vi "點檢_雷射_命令(切圓)VI.vi"(7 "半徑":dbl min=0.0 max=999.0, 8 "error in (no error)":errorcluster, 9 "雷射圓心座標":cluster{"X":dbl, "Y":dbl} {"X" min=0.0 max=220.0}, 10 "掃描速率(刀速)":u16=220 max=2000 format="%0.0f", 11 "功率":u8=70 max=80) -> (0 "error out":errorcluster, 3 "命令字串":string)   [LabVIEW 2015]
panel:
  out "Y座標":string
  out "x座標":string
  out "命令Array":string[](array[string])
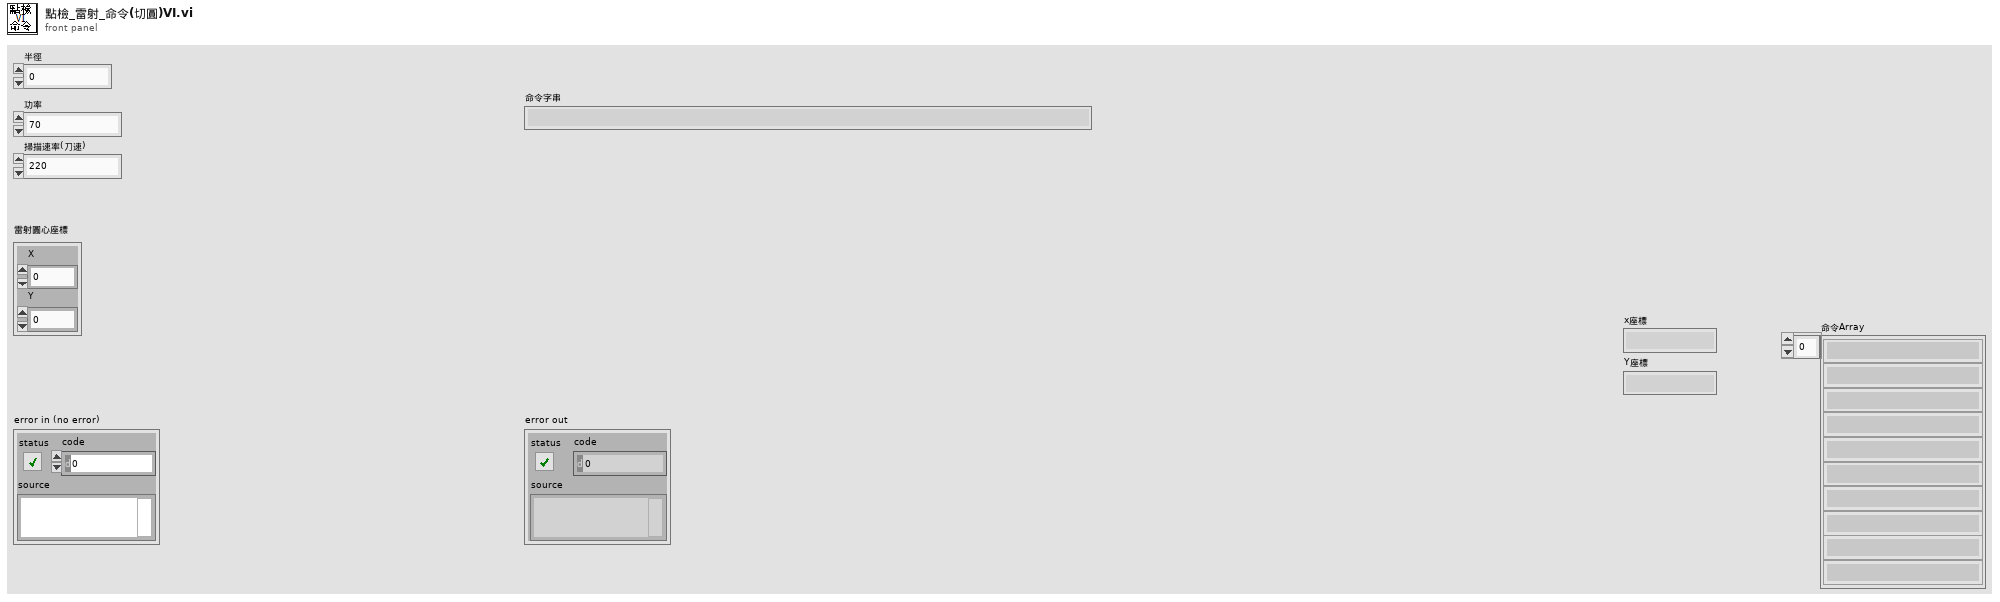
[diagram p1: front panel]
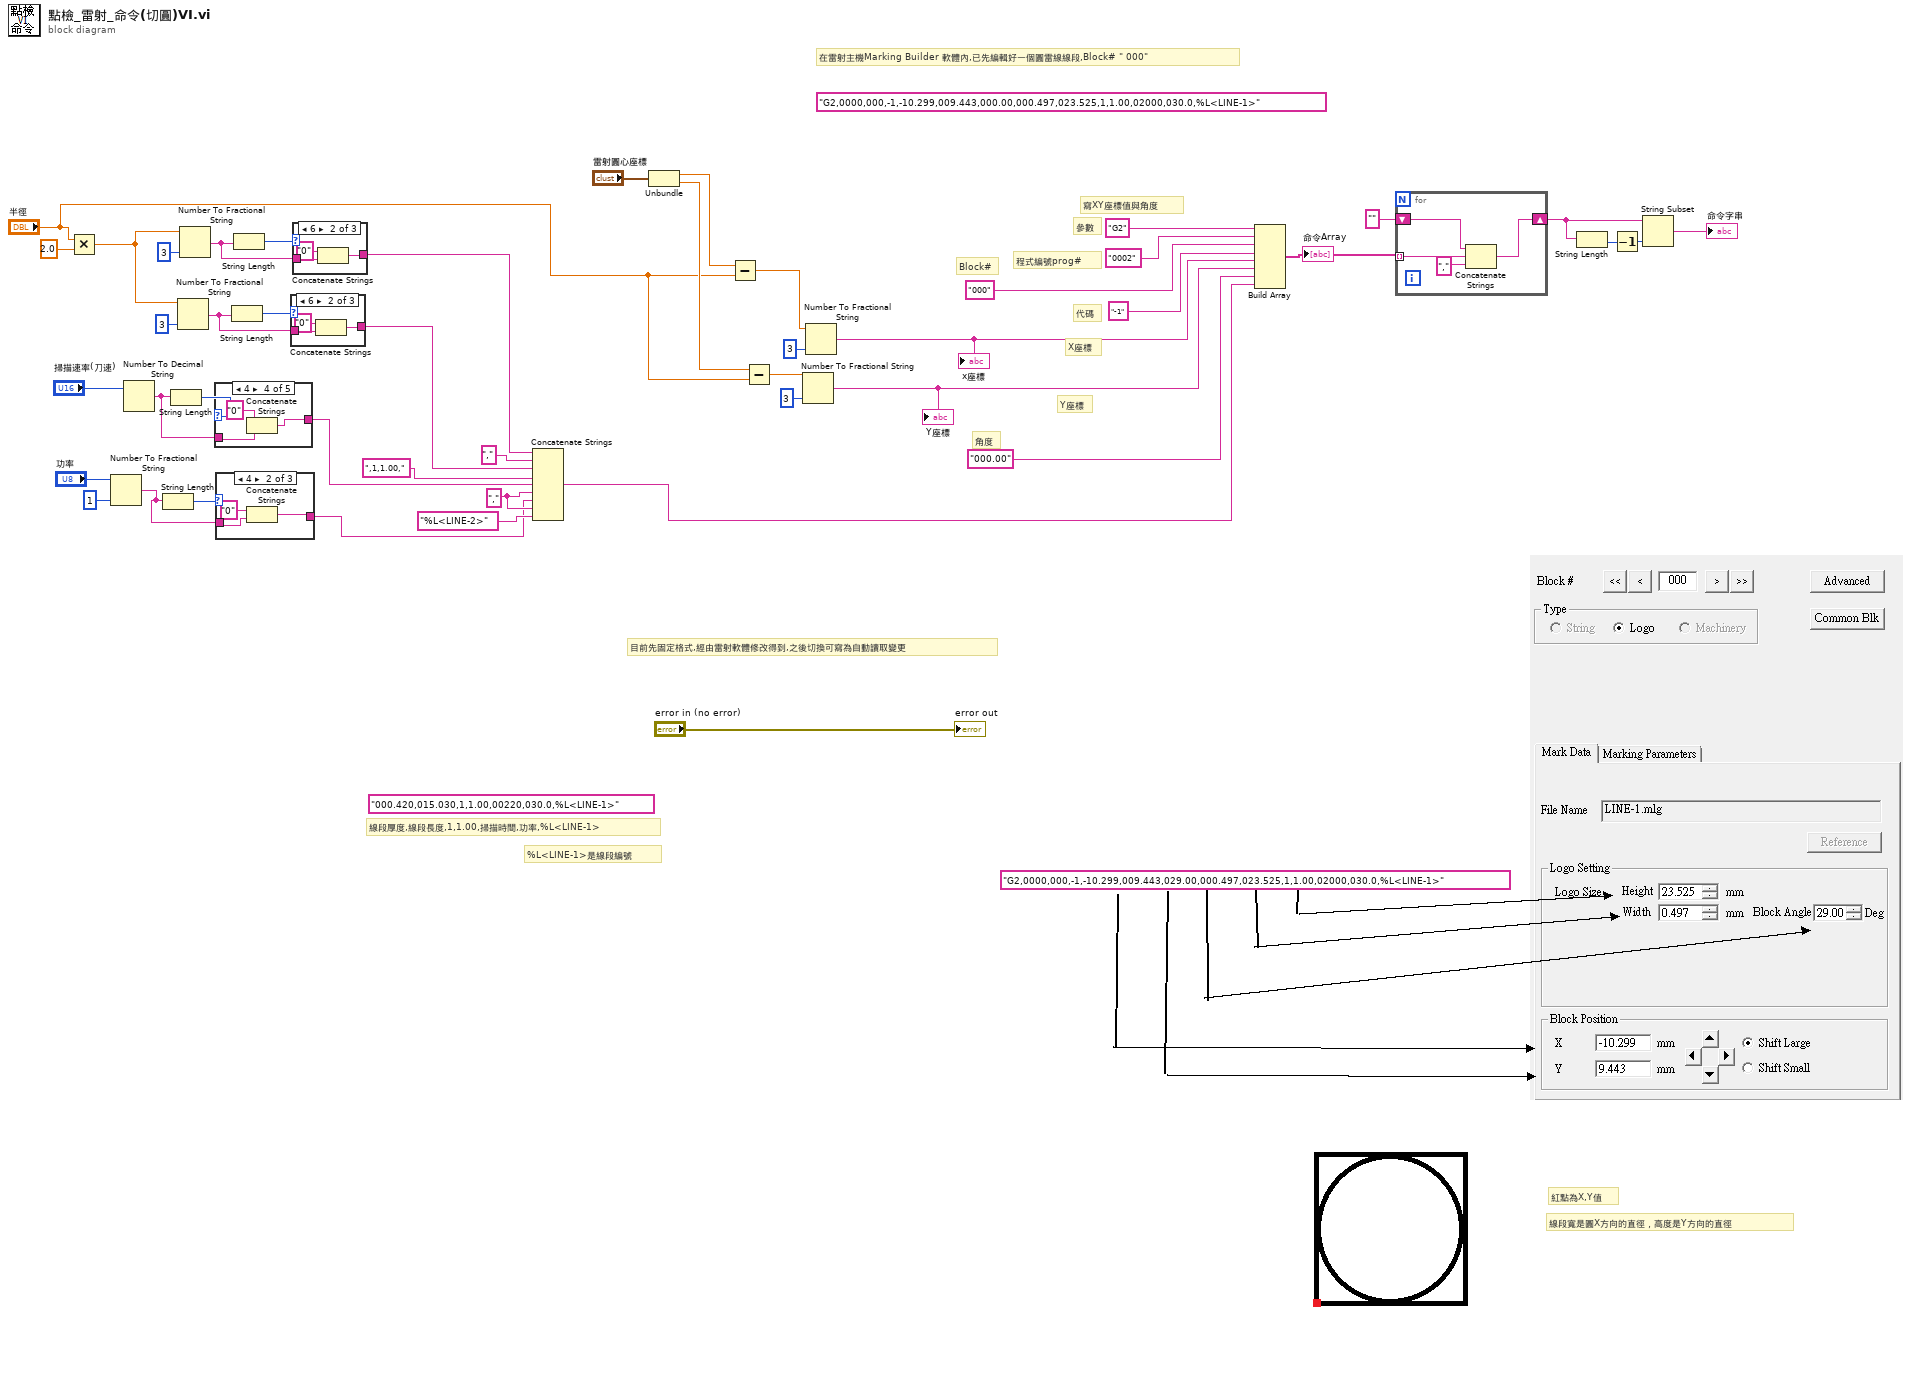
[diagram p0: block diagram]
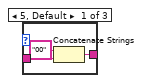
[diagram p2: hidden frame]
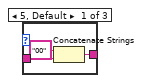
[diagram p4: hidden frame]
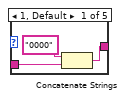
[diagram p6: hidden frame]
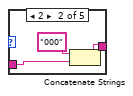
[diagram p7: hidden frame]
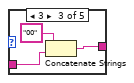
[diagram p8: hidden frame]
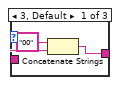
[diagram p10: hidden frame]
diagram:
  w31 = ","
  (unwired) "G2,0000,000,-1,-10.299,009.443,029.00,000.497,023.525,1,1.00,02000,030.0,%L<LINE-1>"
  (unwired) "G2,0000,000,-1,-10.299,009.443,000.00,000.497,023.525,1,1.00,02000,030.0,%L<LINE-1>"
  (unwired) "000.420,015.030,1,1.00,00220,030.0,%L<LINE-1>"
  # "Y座標"
  # "角度"
  # "%L<LINE-1>是線段編號"
  # "線段寬是圓X方向的直徑，高度是Y方向的直徑"
  # "紅點為X,Y值"
  # "Block#"
  # "目前先固定格式,經由雷射軟體修改得到,之後切換可寫為自動讀取變更"
  # "代碼"
  # "在雷射主機Marking Builder 軟體內,已先編輯好一個圓雷線線段,Block# \" 000\""
  # "寫XY座標值與角度"
  # "X座標"
  # "程式編號prog#"
  # "參數"
  # "線段厚度,線段長度,1,1.00,掃描時間,功率,%L<LINE-1>"
  n1 = Multiply(x="半徑", y=2.0) -> (x*y=w9:dbl)
  n2 = Number To Fractional String(number="功率", precision (6)=i16 1 ("width (-)")) -> (F-format string=w27:string)  [unwired: 2 in]
  n3 = Number To Decimal String(number="掃描速率(刀速)") -> (decimal integer string=w29:string)  [unwired: 1 in]
  n4 = String Length(string=w27) -> (length=w26:i32)
  n5 = String Length(string=w29) -> (length=w28:i32)
  n6 = Number To Fractional String(number=w9, precision (6)=i16 3) -> (F-format string=w22:string)  [unwired: 2 in]
  n7 = Number To Fractional String(number=w9, precision (6)=i16 3) -> (F-format string=w12:string)  [unwired: 2 in]
  n8 = case shown="4" w28 {
    tunnel: w29 -> [w49 w51 w55 w57 w59]
    tunnel: [w47 w50 w53 w56 w59] -> w24
    frame 1, Default {
      n9 = Concatenate Strings("0000" ("string"), w49) -> (w47:string)
    }
    frame 2 {
      n10 = Concatenate Strings("000" ("string"), w51) -> (w50:string)
    }
    frame 3 {
      n11 = Concatenate Strings("00" ("string"), w55) -> (w53:string)
    }
    frame 4 {
      n12 = Concatenate Strings("0" ("string"), w57) -> (w56:string)
    }
    frame 5 {
    }
  }
  n13 = case shown="4" w26 {
    tunnel: w27 -> [w62 w64 w66]
    tunnel: [w60 w63 w66] -> w23
    frame 3, Default {
      n14 = Concatenate Strings("00" ("string"), w62) -> (w60:string)
    }
    frame 4 {
      n15 = Concatenate Strings("0" ("string"), w64) -> (w63:string)
    }
    frame 5 {
    }
  }
  n16 = String Length(string=w22) -> (length=w21:i32)
  n17 = String Length(string=w12) -> (length=w13:i32)
  n18 = case shown="6" w21 {
    tunnel: w22 -> [w69 w71 w73]
    tunnel: [w67 w72 w73] -> w19
    frame 5, Default {
      n19 = Concatenate Strings("00" ("string"), w69) -> (w67:string)
    }
    frame 6 {
      n20 = Concatenate Strings("0" ("string"), w71) -> (w72:string)
    }
    frame 7 {
    }
  }
  n21 = case shown="6" w13 {
    tunnel: w12 -> [w76 w78 w80]
    tunnel: [w74 w79 w80] -> w10
    frame 5, Default {
      n22 = Concatenate Strings("00" ("string"), w76) -> (w74:string)
    }
    frame 6 {
      n23 = Concatenate Strings("0" ("string"), w78) -> (w79:string)
    }
    frame 7 {
    }
  }
  n24 = Concatenate Strings(w10, ",", w19, ",1,1.00,", w24, w31, w23, w31, "%L<LINE-2>" ("string")) -> (w35:string)
  n25 = Unbundle("雷射圓心座標") -> ("X"=w6:dbl, "Y"=w3:dbl)
  n26 = Subtract(x=w6, y="半徑") -> (x-y=w5:dbl)
  n27 = Subtract(x=w3, y="半徑") -> (x-y=w4:dbl)
  n28 = Number To Fractional String(number=w4, precision (6)=i16 3) -> (F-format string=w16:string)  [unwired: 2 in]
  "Y座標" <- w16
  n29 = Number To Fractional String(number=w5, precision (6)=i16 3) -> (F-format string=w36:string)  [unwired: 2 in]
  "x座標" <- w36
  n30 = Build Array("G2", "0002", "000", "-1", w36, w16, "000.00", w35) -> (w39:string[])
  "命令Array" <- w39
  n31 = for {
    tunnel: w39 -> [w82] mode=indexing
    shift-right: [w81] -> w44
    shift-left: "" -> [w83]
    n32 = Concatenate Strings(w83, w82, ",") -> (w81:string)
  }
  n33 = String Length(string=w44) -> (length=w45:i32)
  n34 = Decrement(x=w45) -> (x-1=w46:i32)
  n35 = String Subset(string=w44, length (rest)=w46) -> (substring=→"命令字串":string)  [unwired: 1 in]
  "error out" <- "error in (no error)"
